vi "read_config_file.vi"(8 "error in (no error)":errorcluster, 10 "filename":string, 11 "Application Directory":path) -> (0 "error out":errorcluster, 1 "gui_strings":string[](array[string]), 2 "devices":T1, 3 "gral_config":T3={"file_ext"="0.0.0.0", "TCP port"=0, "#devices"=0, "log?"=FALSE, "tcp?"=FALSE, "language"="ENG"})   [LabVIEW 2013]
doc: "Reads the configuration file (config.ini)"
uses:
  <vilib>/Utility/config.llb/NI_LVConfig.lvlib
  <vilib>/Utility/config.llb/Read Key (String).vi
  <vilib>/Utility/config.llb/Read Key (I32).vi
  <vilib>/Utility/config.llb/Read Key (Boolean).vi
  <vilib>/Utility/config.llb/Read Key (Path).vi
  type_def/general.ctl
  type_def/device_array.ctl
  type_def/device.ctl
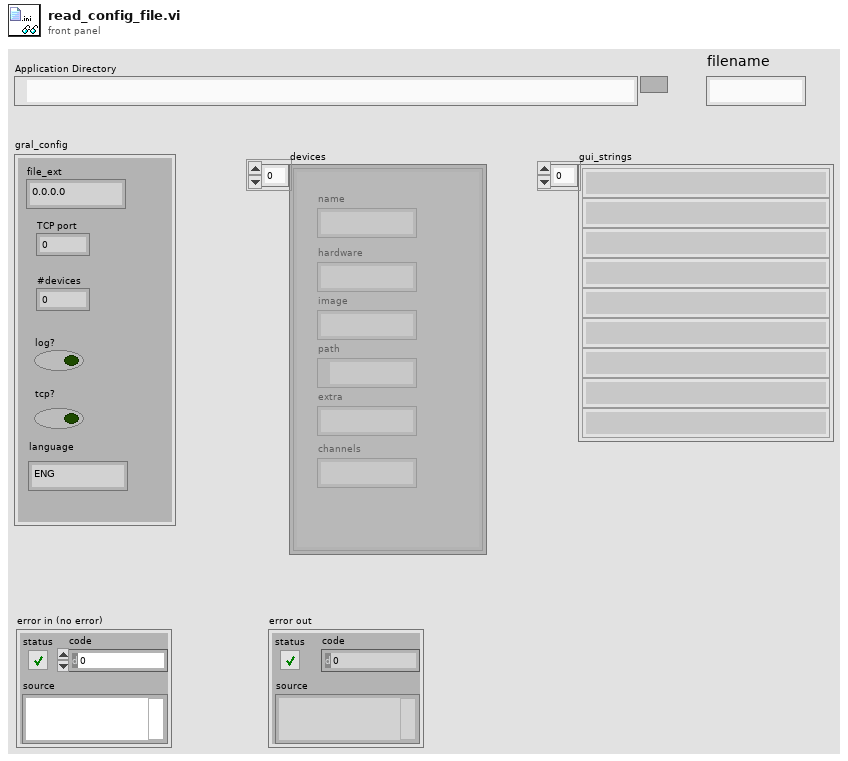
[diagram p1: front panel]
types:
  T1 = typedef "device_array.ctl" = T2[]
  T2 = typedef "device.ctl" = cluster{"name":string, "hardware":string, "image":string, "path":path, "extra":string, "channels":string}
  T3 = typedef "general.ctl" = cluster{"file_ext":string, "TCP port":i32, "#devices":i32, "log?":bool, "tcp?":bool, "language":string}
  T4 = typedef "NI_LVConfig.lvlib/Config Data RefNum.ctl" = refnum<k1>
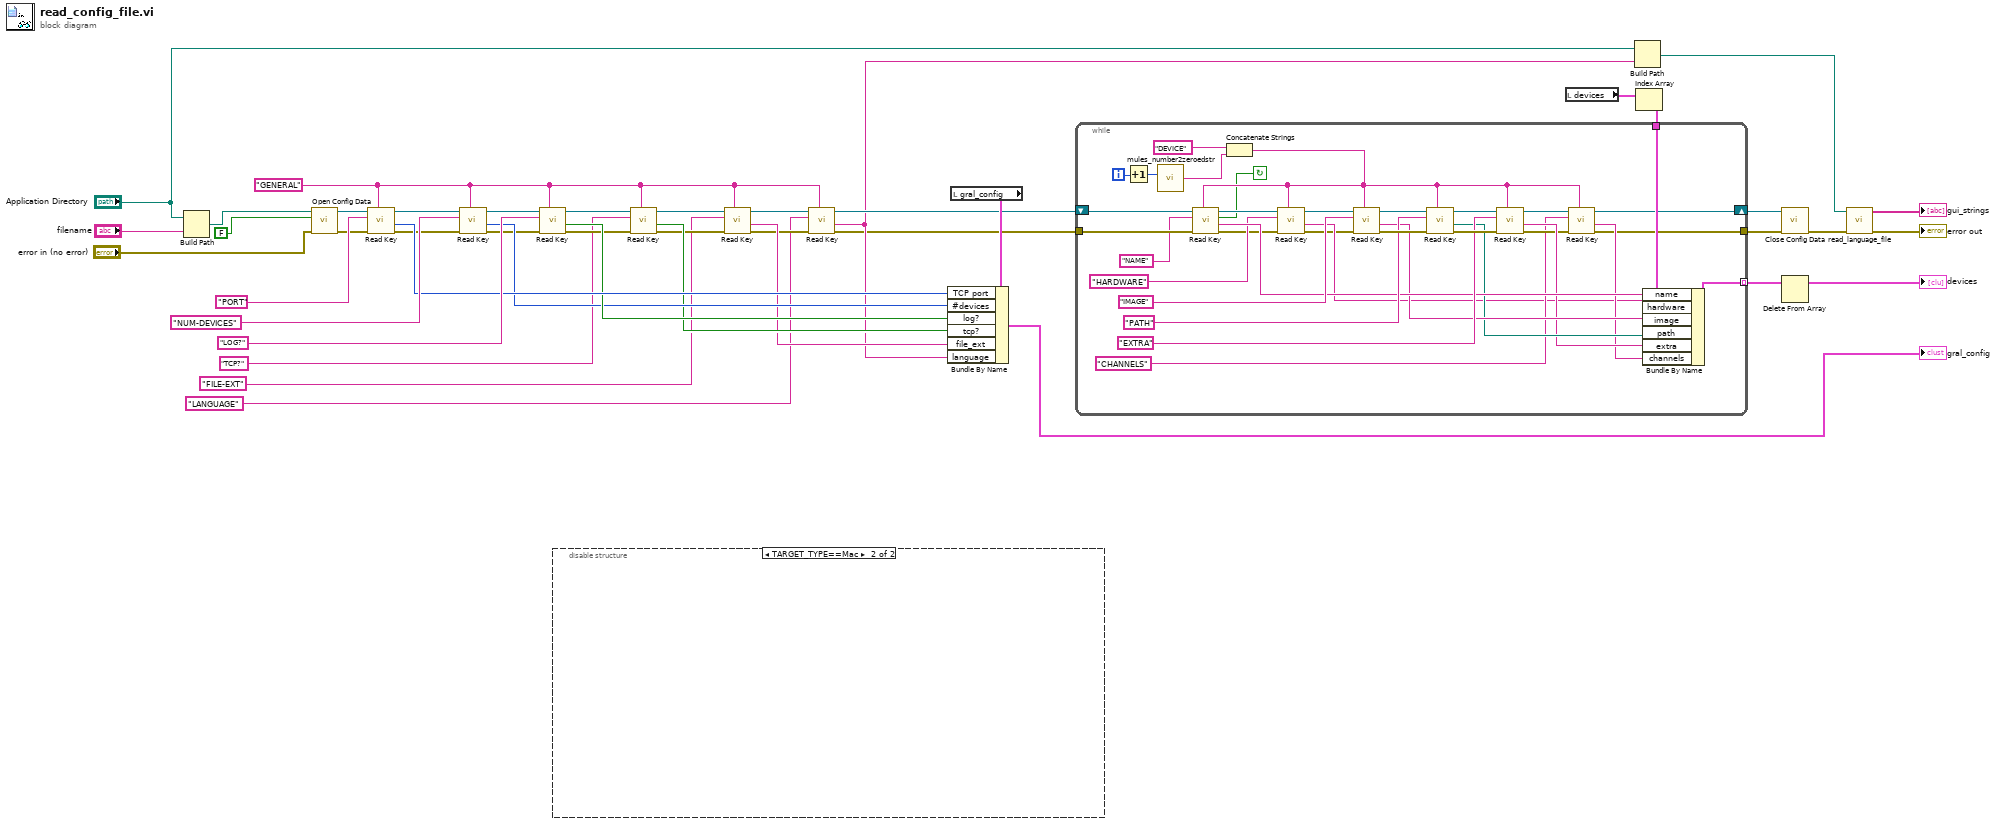
[diagram p0: block diagram]
diagram:
  w18 = "GENERAL" ("section")
  n1 = Build Path(base path="Application Directory", name or relative path="filename") -> (appended path=w44:path)
  n2 = call <vilib>:"Open Config Data.vi"("error in (no error)"="error in (no error)", "create file if necessary (T)"=FALSE, "configuration file path"=w44) -> ("error out"=w11:errorcluster, "refnum"=w14:T4)  [unwired: 6 in, 1 out]
  n3 = call-poly <vilib>:"Read Key.vi"("section"=w18, "error in (no error)"=w11, "key"="PORT", "refnum"=w14) -> ("error out"=w12:errorcluster, "value"=w36:i32, "refnum out"=w13:T4)  [unwired: 4 in, 1 out]
  n4 = call-poly <vilib>:"Read Key.vi"("section"=w18, "error in (no error)"=w12, "key"="NUM-DEVICES", "refnum"=w13) -> ("error out"=w30:errorcluster, "value"=w34:i32, "refnum out"=w40:T4)  [unwired: 4 in, 1 out]
  n5 = call-poly <vilib>:"Read Key.vi"("section"=w18, "error in (no error)"=w30, "key"="LOG?", "refnum"=w40) -> ("error out"=w28:errorcluster, "value"=w35:bool, "refnum out"=w29:T4)  [unwired: 4 in, 1 out]
  n6 = disable-structure shown="TARGET_TYPE==Mac" {
    frame condition #0 {
    }
    frame condition #1 (active) {
    }
  }
  n7 = call-poly <vilib>:"Read Key.vi"("section"=w18, "error in (no error)"=w28, "key"="TCP?", "refnum"=w29) -> ("error out"=w24:errorcluster, "value"=w26:bool, "refnum out"=w25:T4)  [unwired: 4 in, 1 out]
  n8 = call-poly <vilib>:"Read Key.vi"("section"=w18, "error in (no error)"=w24, "key"="FILE-EXT", "refnum"=w25) -> ("error out"=w21:errorcluster, "value"=w22:string, "refnum out"=w19:T4)  [unwired: 4 in, 1 out]
  n9 = call-poly <vilib>:"Read Key.vi"("section"=w18, "error in (no error)"=w21, "key"="LANGUAGE", "refnum"=w19) -> ("error out"=w4:errorcluster, "value"=w9:string, "refnum out"=w20:T4)  [unwired: 4 in, 1 out]
  n10 = local read "gral_config"() -> (w37:T3)
  n11 = Bundle By Name(cluster=w37, "TCP port"=w36, "#devices"=w34, "log?"=w35, "tcp?"=w26, "file_ext"=w22, "language"=w9) -> (→"gral_config":T3)
  n12 = local read "devices"() -> (w33:T1)
  n13 = Build Path(base path="Application Directory", name or relative path=w9) -> (appended path=w10:path)
  n14 = Index Array(array=w33) -> (element=w32:T2)  [unwired: 1 in]
  n15 = while {
    shift-right: [w57] -> w41
    shift-left: w20 -> [w76]
    tunnel: w32 -> [w64]
    tunnel: [w63] -> w16 mode=indexing
    tunnel: w4 -> [w71]
    tunnel: [w45] -> w3
    i -> [w78]
    stop <- w46 continue-if-true
    n16 = Increment(x=w78) -> (x+1=w77:i32)
    n17 = call "mules_number2zeroedstr.vi"("number"=w77) -> ("string"=w65:string)  [unwired: 1 in]
    n18 = Concatenate Strings("DEVICE" ("key"), w65) -> (w51:string)
    n19 = call-poly <vilib>:"Read Key.vi"("section"=w51, "error in (no error)"=w71, "key"="NAME", "refnum"=w76) -> ("error out"=w48:errorcluster, "value"=w62:string, "found?"=w46:bool, "refnum out"=w53:T4)  [unwired: 4 in]
    n20 = call-poly <vilib>:"Read Key.vi"("section"=w51, "error in (no error)"=w48, "key"="HARDWARE", "refnum"=w53) -> ("error out"=w47:errorcluster, "value"=w49:string, "refnum out"=w52:T4)  [unwired: 4 in, 1 out]
    n21 = call-poly <vilib>:"Read Key.vi"("section"=w51, "error in (no error)"=w47, "key"="IMAGE", "refnum"=w52) -> ("error out"=w72:errorcluster, "value"=w61:string, "refnum out"=w75:T4)  [unwired: 4 in, 1 out]
    n22 = call-poly <vilib>:"Read Key.vi"("section"=w51, "error in (no error)"=w72, "key"="PATH", "refnum"=w75) -> ("error out"=w73:errorcluster, "value"=w60:path, "refnum out"=w74:T4)  [unwired: 4 in, 1 out]
    n23 = call-poly <vilib>:"Read Key.vi"("section"=w51, "error in (no error)"=w73, "key"="EXTRA", "refnum"=w74) -> ("error out"=w58:errorcluster, "value"=w59:string, "refnum out"=w56:T4)  [unwired: 4 in, 1 out]
    n24 = call-poly <vilib>:"Read Key.vi"("section"=w51, "error in (no error)"=w58, "key"="CHANNELS", "refnum"=w56) -> ("error out"=w45:errorcluster, "value"=w54:string, "refnum out"=w57:T4)  [unwired: 4 in, 1 out]
    n25 = Bundle By Name(cluster=w64, "name"=w62, "hardware"=w49, "image"=w61, "path"=w60, "extra"=w59, "channels"=w54) -> (w63:T2)
  }
  n26 = call <vilib>:"Close Config Data.vi"("error in (no error)"=w3, "refnum"=w41) -> ("error out"=w2:errorcluster)  [unwired: 8 in, 1 out]
  n27 = Delete From Array(array=w16) -> (array with subset deleted=→"devices":T2[])  [unwired: 2 in, 1 out]
  n28 = call "read_language_file.vi"("error in"=w2, "Text File"=w10) -> ("error out"=→"error out":errorcluster, "gui_strings"=→"gui_strings":string[])  [unwired: 8 in]
